vi "Untitled 3.vi"(8 "error in":errorcluster, 11 "Class 2 in":refnum<class "Class 2.lvclass">) -> (0 "error out":errorcluster, 3 "Class 2 out":refnum<class "Class 2.lvclass">)   [LabVIEW 2020, in "Class 2.lvclass"]
uses:
  Class 2.lvclass
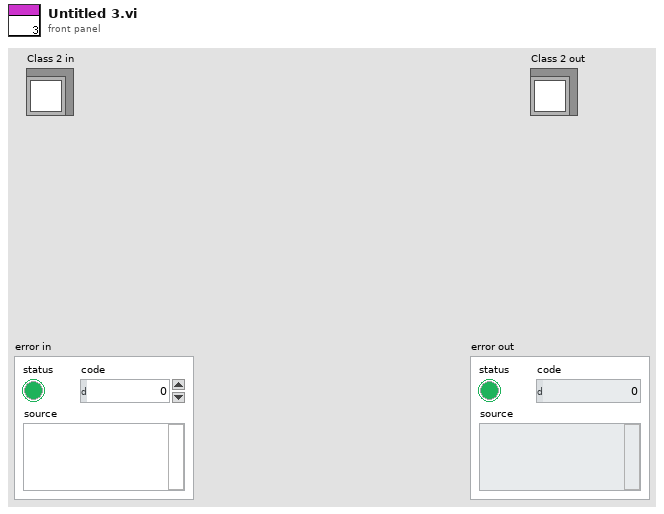
[diagram p1: front panel]
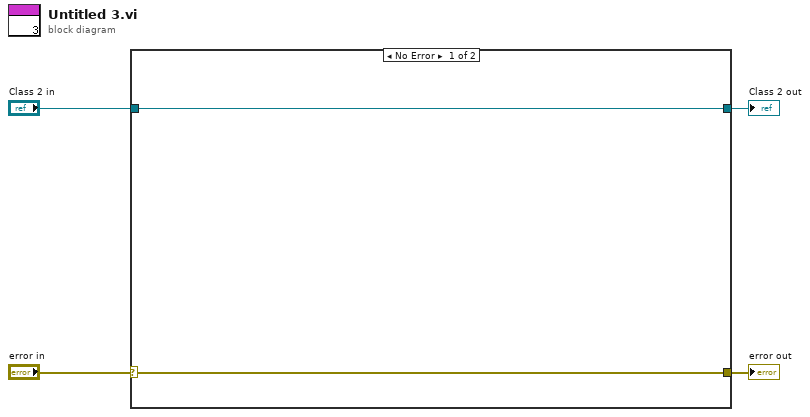
[diagram p0: block diagram]
diagram:
  n1 = case shown="No Error" "error in" {
    selector: "error in" -> [w5 w8]
    tunnel: [w5 w8] -> w1
    tunnel: [w6 w7] -> w3
    tunnel: "Class 2 in" -> [w6 w7]
    frame No Error {
    }
    frame Error {
    }
  }
  "Class 2 out" <- w3
  "error out" <- w1
